vi "Write Data.vi"(6 "Unit ID":u8, 7 "Write Mask":bool[](array[boolean]), 8 "error in (no error)":errorcluster, 9 "Values":dbl[](array[numeric]), 10 "output data access":T1={"Modbus Type"=enum."Input Register", "start"=0, "length"=0, "Channel Data"=[]}, 11 "Modbus Master in":refnum<class "Modbus Master.lvclass">) -> (0 "error out":errorcluster)   [LabVIEW 2015, in "Modbus Master Engine.lvlib"]
uses:
  Modbus Master Engine.lvlib
  Modbus API.lvlibp/API/Master/Modbus Master.lvclass
  Bulk Data Access.ctl
  System Explorer/SubVIs/Modbus Type.ctl
  Shared/Controls/Data Model/Channel.ctl
  <vilib>/NI Veristand/Custom Device API/Custom Device Channel Type.ctl
  Shared/Controls/Data Model/Mapping.ctl
  Shared/Controls/Data Model/DataType.ctl
  <vilib>/NI Veristand/Custom Device API/Custom Device Item Ref.ctl
  Shared/Modbus Master Shared.lvlib
  <vilib>/NI VeriStand/Custom Device API/Custom Device API.lvlib
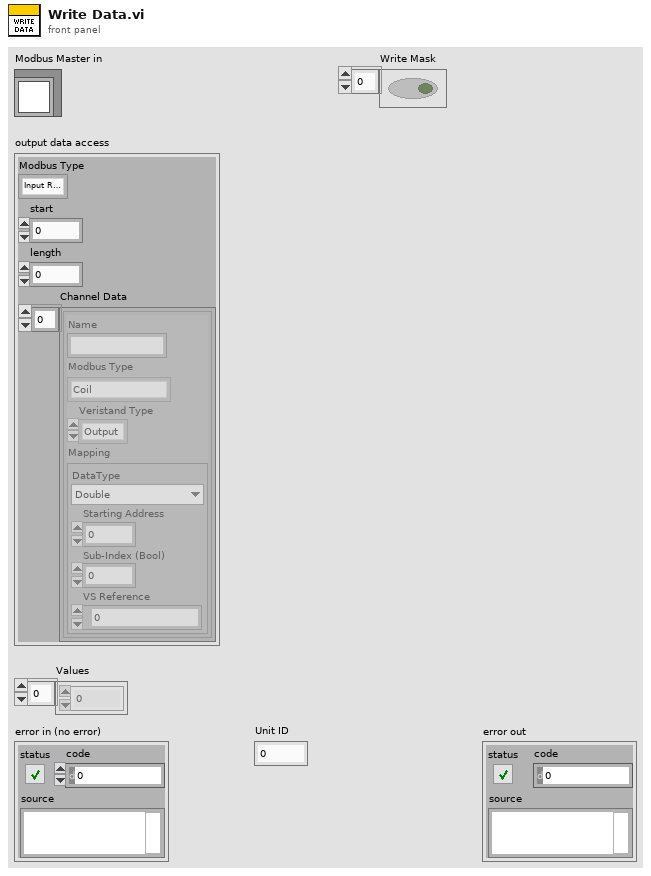
[diagram p1: front panel]
types:
  T1 = typedef "Modbus Master Shared.lvlib/Bulk Data Access.ctl" = cluster{"Modbus Type":T2, "start":u16, "length":u16, "Channel Data":T3[]}
  T2 = typedef "Modbus Master Shared.lvlib/Modbus Type.ctl" = enum16{"Coil", "Discrete Input", "Holding Register", "Input Register"}
  T3 = typedef "Modbus Master Shared.lvlib/Channel.ctl" = cluster{"Name":string, "Modbus Type":T2, "Veristand Type":T4, "Mapping":T5}
  T4 = typedef "Custom Device API.lvlib/Custom Device Channel Type.ctl" = enum16{"Input", "Output"}
  T5 = typedef "Modbus Master Shared.lvlib/Mapping.ctl" = cluster{"DataType":T6, "Starting Address":u16, "Sub-Index (Bool)":u16, "VS Reference":T7}
  T6 = typedef "Modbus Master Shared.lvlib/DataType.ctl" = enum16{"Double", "Single", "I64", "I32", "I16", "I8", "U64", "U32", "U16", "U8", "Boolean"}
  T7 = typedef "Custom Device API.lvlib/Custom Device Item Ref.ctl" = u64
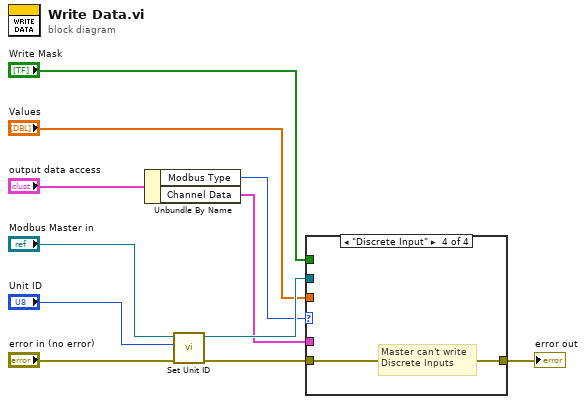
[diagram p0: block diagram]
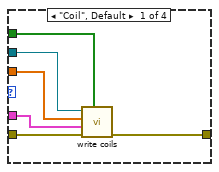
[diagram p2: hidden frame]
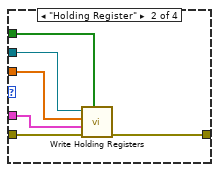
[diagram p3: hidden frame]
diagram:
  n1 = Unbundle By Name("output data access") -> ("Modbus Type"=w2:T2, "Channel Data"=w1:T3[])
  n2 = call "Set Unit ID.vi"("error in"="error in (no error)", "unit ID"="Unit ID", "Modbus master in"="Modbus Master in") -> ("error out"=w11:errorcluster, "Modbus master out"=w8:refnum<class "Modbus Master.lvclass">)  [unwired: 7 in]
  n3 = case shown="\"Discrete Input\"" w2 {
    tunnel: w8 -> [w12 w23 _ _]
    tunnel: [w17 w22 w24 w25] -> w4
    tunnel: w11 -> [w16 w21 w24 w25]
    tunnel: w1 -> [w13 w20 _ _]
    tunnel: "Write Mask" -> [w15 w19 _ _]
    tunnel: "Values" -> [w14 w18 _ _]
    frame "Coil", Default {
      n4 = call "write coils.vi"("Array"=w15, "error in (no error)"=w16, "Channel Data"=w13, "Values"=w14, "Modbus API.lvlibp:Modbus API"=w12) -> ("error out"=w17:errorcluster)  [unwired: 6 in]
    }
    frame "Holding Register" {
      n5 = call "Write Holding Registers.vi"("Regs to Write"=w19, "error in (no error)"=w21, "Channel Data"=w20, "Values"=w18, "Modbus API.lvlibp:Modbus API"=w23) -> ("error out"=w22:errorcluster)  [unwired: 6 in]
    }
    frame "Input Register" {
      # "Master can't write\nInput Regs"
    }
    frame "Discrete Input" {
      # "Master can't write\nDiscrete Inputs"
    }
  }
  "error out" <- w4
